vi "toml_lock_obtain.vi"(8 "error in (no error)":errorcluster, 11 "path in":path) -> (0 "error out":errorcluster, 1 "locks":refnum<queue>[](array[refnum]), 2 "resolved path":path, 3 "lock":refnum<queue>)   [LabVIEW 2017]
uses:
  <vilib>/Utility/file.llb/Application Directory.vi
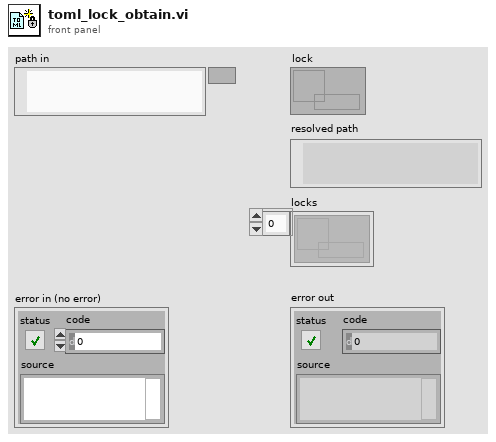
[diagram p1: front panel]
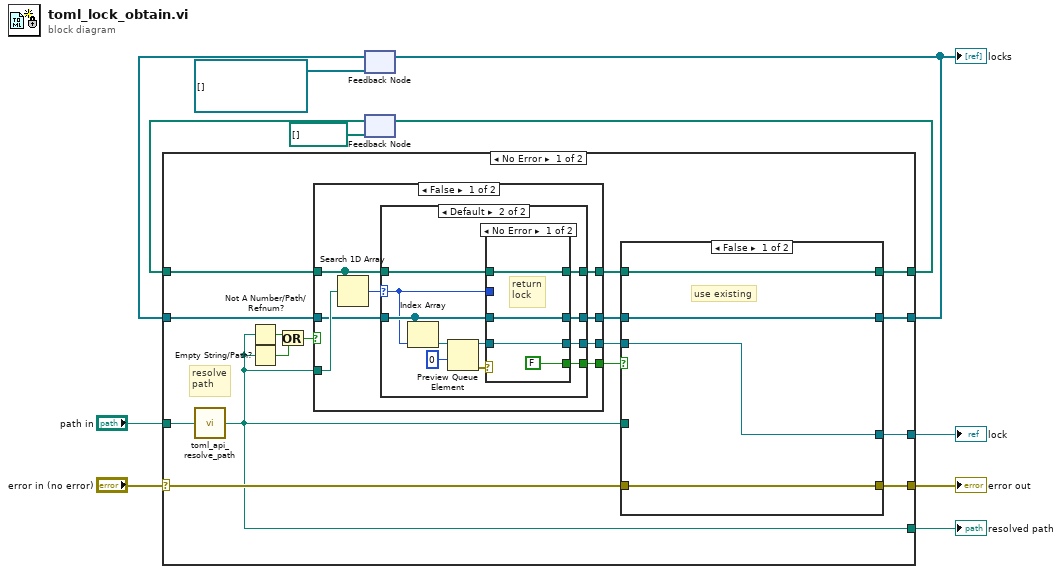
[diagram p0: block diagram]
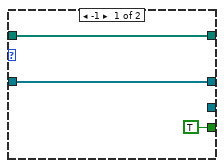
[diagram p2: hidden frame]
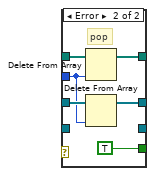
[diagram p3: hidden frame]
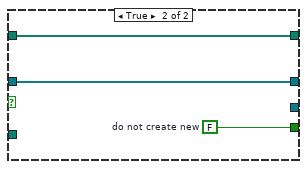
[diagram p4: hidden frame]
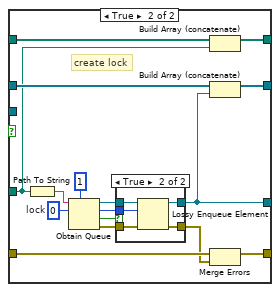
[diagram p5: hidden frame]
diagram:
  n1 = feedback #1(refnum<queue>[] []) -> (w2:refnum<queue>[])
  n2 = feedback #2(path[] []) -> (w3:path[])
  n3 = case shown="No Error" "error in (no error)" {
    selector: "error in (no error)" -> [w25 w91]
    tunnel: "path in" -> [w27 _]
    tunnel: [w26 w91] -> w1
    tunnel: [w24 _] -> w9
    tunnel: [w23 w89] -> w6
    tunnel: [w22 w90] -> w5
    tunnel: [w15 _] -> w4
    tunnel: w3 -> [w20 w90]
    tunnel: w2 -> [w18 w89]
    frame No Error {
      # "resolve\npath"
      n4 = call "toml_api_resolve_path.vi"("path"=w27) -> ("resolved path"=w15:path)
      n5 = Not A Number/Path/Refnum?(number/path/refnum=w15) -> (NaN/Path/Refnum?=w14:bool)
      n6 = Empty String/Path?(string/path=w15) -> (empty?=w13:bool)
      n7 = Or(x=w14, y=w13) -> (x .or. y?=w12:bool)
      n8 = case shown="False" w12 {
        tunnel: w15 -> [w35 _]
        tunnel: [w34 w61] -> w21
        tunnel: w20 -> [w33 w61]
        tunnel: [w32 w62] -> w19
        tunnel: w18 -> [w31 w62]
        tunnel: [w29 w60] -> w17
        tunnel: [w28 _] -> w16
        frame False {
          n9 = Search 1D Array(1D array=w33, element=w35) -> (index of element=w30:i32)  [unwired: 1 in]
          n10 = case shown="Default" w30 {
            selector: w30 -> [_ w42]
            tunnel: [w38 w49] -> w34
            tunnel: w33 -> [w38 w48]
            tunnel: [w37 w47] -> w32
            tunnel: w31 -> [w37 w46]
            tunnel: [TRUE w41] -> w29
            tunnel: [_ w40] -> w28
            frame -1 {
            }
            frame Default {
              n11 = Index Array(array=w46, index=w42) -> (element=w45:refnum<queue>)
              n12 = Preview Queue Element(queue=w45, timeout in ms (-1)=0) -> (queue out=w39:refnum<queue>, error out=w43:errorcluster)  [unwired: 1 in, 2 out]
              n13 = case shown="No Error" w43 {
                tunnel: [w51 w59] -> w49
                tunnel: w48 -> [w51 w58]
                tunnel: [w52 w57] -> w47
                tunnel: w46 -> [w52 w56]
                tunnel: w42 -> [_ w55]
                tunnel: [FALSE TRUE] -> w41
                tunnel: [w53 _] -> w40
                tunnel: w39 -> [w53 _]
                frame No Error {
                  # "return\nlock"
                }
                frame Error {
                  # "pop"
                  n14 = Delete From Array(array=w58, index=w55) -> (array with subset deleted=w59:path[])  [unwired: 1 in, 1 out]
                  n15 = Delete From Array(array=w56, index=w55) -> (array with subset deleted=w57:refnum<queue>[])  [unwired: 1 in, 1 out]
                }
              }
            }
          }
        }
        frame True {
          w60 = FALSE  # do not create new
        }
      }
      n16 = case shown="False" w17 {
        tunnel: [w66 w81] -> w26
        tunnel: w25 -> [w66 w80]
        tunnel: w15 -> [_ w68]
        tunnel: [w65 w67] -> w24
        tunnel: [w64 w69] -> w23
        tunnel: w19 -> [w64 w72]
        tunnel: [w63 w70] -> w22
        tunnel: w21 -> [w63 w71]
        tunnel: w16 -> [w65 _]
        frame False {
          # "use existing"
        }
        frame True {
          w77 = u8 0  # lock
          # "create lock"
          n17 = Path To String(path=w68) -> (string=w74:string)
          n18 = Obtain Queue(max queue size (-1, unlimited)=1, name (unnamed)=w74, element data type=w77) -> (queue out=w76:refnum<queue>, created new?=w79:bool, error out=w78:errorcluster)  [unwired: 2 in]
          n19 = case shown="True" w79 {
            tunnel: w76 -> [w83 w88]
            tunnel: w77 -> [_ w87]
            tunnel: w78 -> [w82 w86]
            tunnel: [w83 w85] -> w67
            tunnel: [w82 w84] -> w73
            frame False {
            }
            frame True {
              n20 = Lossy Enqueue Element(queue=w88, element=w87, error in (no error)=w86) -> (queue out=w85:refnum<queue>, error out=w84:errorcluster)  [unwired: 2 out]
            }
          }
          n21 = Build Array (concatenate)(w71, w68) -> (w70:path[])
          n22 = Build Array (concatenate)(w72, w67) -> (w69:refnum<queue>[])
          n23 = Merge Errors(w80, w73) -> (w81:errorcluster)
        }
      }
    }
    frame Error {
    }
  }
  "lock" <- w9
  "resolved path" <- w4
  "locks" <- w6
  "error out" <- w1
  n24 = feedback-in #1(w6) -> ()
  n25 = feedback-in #2(w5) -> ()
